vi "Junk.vi"() -> ()   [LabVIEW 2017]
uses:
  <vilib>/Analysis/baseanly.llb/Mean (DBL).vi
  <vilib>/Analysis/NI_AALBase.lvlib
panel:
  in  "Tab Control":enum32{"MIN", "MAX", "SP", "RMS"}(tab)
  in  "MIN Array":bool[](array[boolean])
  in  "MAX Array":bool[](array[boolean])
  in  "SP Array":bool[](array[boolean])
  in  "RMS Array":bool[](array[boolean])
  in  "Array-RMS":refnum<vi>
  in  "Array-SP":refnum<vi>
  in  "Array-MAX":refnum<vi>
  in  "Array-MIN":refnum<vi>
  in  "Array":bool[](array[boolean])
  out "Avilable Wfms":string[](array[string])
  in  "Avalable Wfms":string[](array[string])
  in  "Prevoiusly Selected Wfms":string[](array[string])
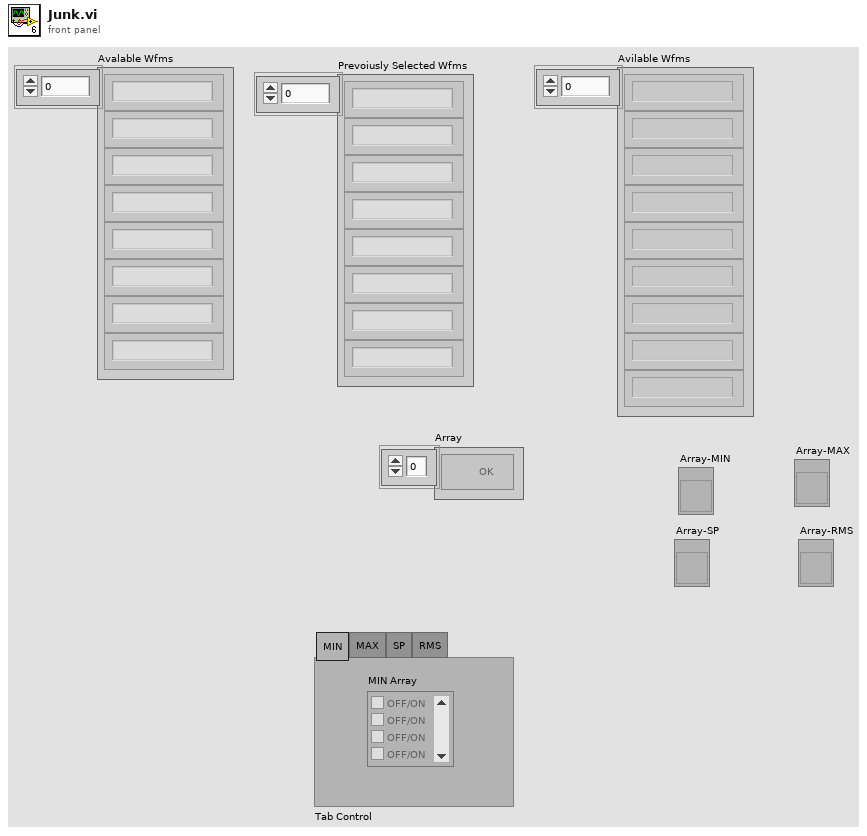
[diagram p1: front panel]
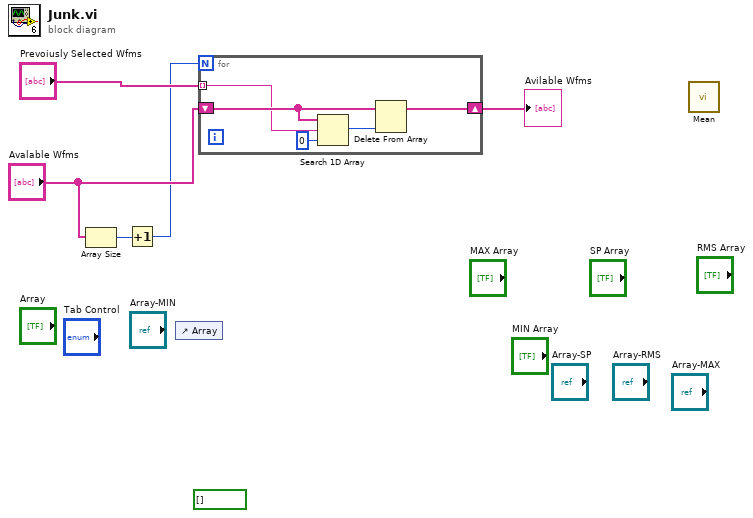
[diagram p0: block diagram]
diagram:
  (unwired) bool[] []
  n1 = Array Size(array="Avalable Wfms") -> (size(s)=w2:i32)
  n2 = Increment(x=w2) -> (x+1=w1:i32)
  n3 = control-ref of="Array"() -> ()  [unwired: 1 out]
  n4 = for {
    N: w1 -> [_]
    tunnel: "Prevoiusly Selected Wfms" -> [w8] mode=indexing
    shift-right: [w9] -> w4
    shift-left: "Avalable Wfms" -> [w10]
    n5 = Search 1D Array(1D array=w10, element=w8, start index (0)=0) -> (index of element=w6:i32)
    n6 = Delete From Array(array=w10, index=w6) -> (array with subset deleted=w9:string[])  [unwired: 1 in, 1 out]
  }
  "Avilable Wfms" <- w4
  n7 = call-poly <vilib>:"Mean.vi"() -> ()  [unwired: 1 in, 2 out]
